vi "Check Sample Container.vi"(8 "error in (no error)":errorcluster, 10 "Sample Container":T1, 11 "CO2 Actor in":refnum<class "CO2 Actor.lvclass">) -> (0 "error out":errorcluster, 3 "CO2 Actor out":refnum<class "CO2 Actor.lvclass">)   [LabVIEW 2015, in "cRIO-Carbondioxide.lvlib" / "CO2-Actor.lvlib" / "CO2 Actor.lvclass"]
uses:
  CO2 Actor.lvclass
  Controls/Sample Container.ctl
  subs/Sample/Sample.lvclass
  <vilib>/ActorFramework/Actor/Actor.lvclass/Actor.ctl
  <vilib>/ActorFramework/Message Enqueuer/Message Enqueuer.lvclass/Message Enqueuer.ctl
  Transfer Line Messages/Sample In Msg/Sample In Msg.lvclass/Sample In Msg.ctl
  <vilib>/ActorFramework/Actor/Read Self Enqueuer.vi
  <vilib>/ActorFramework/Message Enqueuer/Enqueue.vi
  <vilib>/ActorFramework/Message Enqueuer/Init from Existing Queue.vi
  <vilib>/ActorFramework/Message Priority Queue/Priority Enqueue.vi
  <vilib>/ActorFramework/Actor/Actor.lvclass
  <vilib>/ActorFramework/Message Enqueuer/Message Enqueuer.lvclass
  Transfer Line Messages/Sample In Msg/Sample In Msg.lvclass
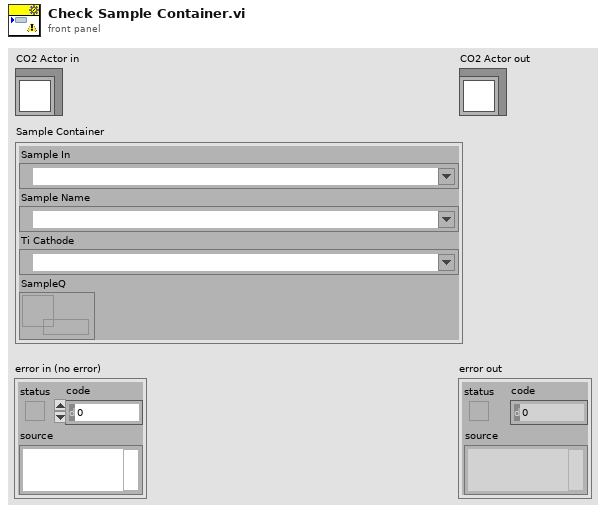
[diagram p1: front panel]
types:
  T1 = typedef "Sample Container.ctl" = cluster{"Sample In":refnum<k21>, "Sample Name":refnum<k21>, "Ti Cathode":refnum<k21>, "SampleQ":refnum<queue>}
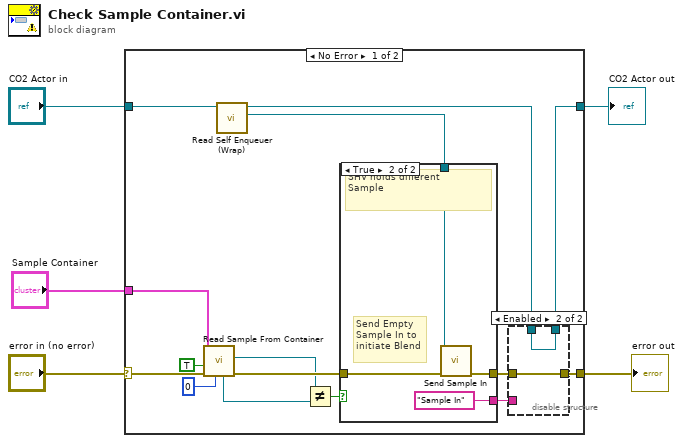
[diagram p0: block diagram]
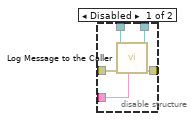
[diagram p2: hidden frame]
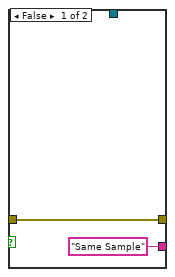
[diagram p3: hidden frame]
diagram:
  n1 = case shown="No Error" "error in (no error)" {
    selector: "error in (no error)" -> [w11 w35]
    tunnel: [w18 w35] -> w4
    tunnel: "Sample Container" -> [w14 _]
    tunnel: "CO2 Actor in" -> [w9 w34]
    tunnel: [w6 w34] -> w1
    frame No Error {
      n2 = call "Read Sample From Container.vi"("Queue timeout in ms (-1)"=0, "error in (no error)"=w11, "Read from SHV (F)"=TRUE, "Container"=w14) -> ("error out"=w12:errorcluster, "Sample out"=w10:refnum<class "Sample.lvclass">, "Overflow Sample"=w15:refnum<class "Sample.lvclass">)  [unwired: 3 in, 2 out]
      n3 = call "Read Self Enqueuer (Wrap).vi"("CO2 Actor in"=w9) -> ("Actor Framework:Message Enqueuer"=w8:refnum<class "Message Enqueuer.lvclass">, "CO2 Actor out"=w7:refnum<class "CO2 Actor.lvclass">)  [unwired: 9 in]
      n4 = Not Equal?(x=w10, y=w15) -> (x != y?=w17:bool)
      n5 = case shown="True" w17 {
        tunnel: w12 -> [w29 w33]
        tunnel: w8 -> [_ w32]
        tunnel: [w29 w31] -> w19
        tunnel: ["Same Sample" ("String (\"\" = no message to send)") "Sample In" ("String (\"\" = no message to send)")] -> w16
        frame False {
        }
        frame True {
          # "Send Empty \nSample In to\ninitiate Blend"
          # "SHV holds different\nSample"
          n6 = call "Send Sample In.vi"("error in (no error)"=w33, "Message Enqueuer"=w32) -> ("error out"=w31:errorcluster)  [unwired: 8 in, 1 out]
        }
      }
      n7 = disable-structure shown="Enabled" {
        disable-tunnel: w19 -> [w25 w27]
        disable-tunnel: [w24 w27] -> w18
        disable-tunnel: w7 -> [w23 w26]
        disable-tunnel: w16 -> [w22 _]
        disable-tunnel: [w21 w26] -> w6
        frame Disabled {
          n8 = call-dynamic "Log Message to the Caller.vi"("String (\"\" = no message to send)"=w22, "error in (no error)"=w25, "CO2 Actor in"=w23) -> ("error out"=w24:errorcluster, "CO2 Actor out"=w21:refnum<class "CO2 Actor.lvclass">)  [unwired: 7 in]
        }
        frame Enabled {
        }
      }
    }
    frame Error {
    }
  }
  "error out" <- w4
  "CO2 Actor out" <- w1
